vi "函数类型1测试.vi"() -> ()   [LabVIEW 2010]
uses:
  全局量/试验配置信息.vi
  全局量/全局_配置.vi
panel:
  out "D_IN_1":string[][](table) caption="表格"
  in  "加载文件名称":string
  out "配置文件路径":path
  out "配置文件目录":path
  in  "加载配置文件列表":u16(ring)
  in  "同步_1":i32
  in  "数组_反馈值":dbl[][](array[numeric])
  in  "第几个数据":i32
  in  "第几组数据":i32
  out "数组_AD幅值":sgl[](array[numeric])
  out "数组_DSP幅值":sgl[](array[numeric])
  in  "数组_设定值":dbl[][](array[numeric])
  in  "数组_选择":bool[](array[boolean])
  out "light_32":bool
  out "light_31":bool
  out "light_30":bool
  out "light_29":bool
  out "light_28":bool
  out "light_27":bool
  out "light_26":bool
  out "light_25":bool
  out "light_24":bool
  out "light_23":bool
  out "light_22":bool
  out "light_21":bool
  out "light_20":bool
  out "light_19":bool
  out "light_18":bool
  out "light_17":bool
  out "Analog_back":string[][](table) caption="表格"
  in  "A_32":bool
  in  "A_31":bool
  in  "A_30":bool
  in  "A_29":bool
  in  "A_28":bool
  in  "A_27":bool
  in  "A_26":bool
  in  "A_25":bool
  in  "A_24":bool
  in  "A_23":bool
  in  "A_22":bool
  in  "A_21":bool
  in  "A_20":bool
  in  "A_19":bool
  in  "A_18":bool
  in  "A_17":bool
  out "合格？":bool[][](array[boolean])
  out "测试结论":string
  out "light_16":bool
  out "light_15":bool
  out "light_14":bool
  out "light_13":bool
  out "light_12":bool
  out "light_11":bool
  out "light_10":bool
  out "light_9":bool
  out "light_8":bool
  out "light_7":bool
  out "light_6":bool
  out "light_5":bool
  out "light_4":bool
  out "light_3":bool
  out "light_2":bool
  out "light_1":bool
  out "退出？":bool
  in  "btn_反选":bool
  in  "btn_全选":bool
  in  "A_16":bool
  in  "A_15":bool
  in  "A_14":bool
  in  "A_13":bool
  in  "A_12":bool
  in  "A_11":bool
  in  "A_10":bool
  in  "A_9":bool
  in  "A_8":bool
  in  "A_7":bool
  in  "A_6":bool
  in  "A_5":bool
  in  "A_4":bool
  in  "A_3":bool
  in  "A_2":bool
  in  "A_1":bool
  in  "btn_取消":bool
  in  "btn_开始测试":bool
  in  "Analog_IN":string[][](table) caption="表格"
  out "Analog_WC":string[][](table) caption="表格"
  # "模拟量选择及输入值（V）"
  # "模拟量反馈值（V）"
  # "模拟量误差值（%）"
  # "加载配置文件："
  # "测试结论："
  # "从0开始"
  # "从1开始,第0列没有使用"
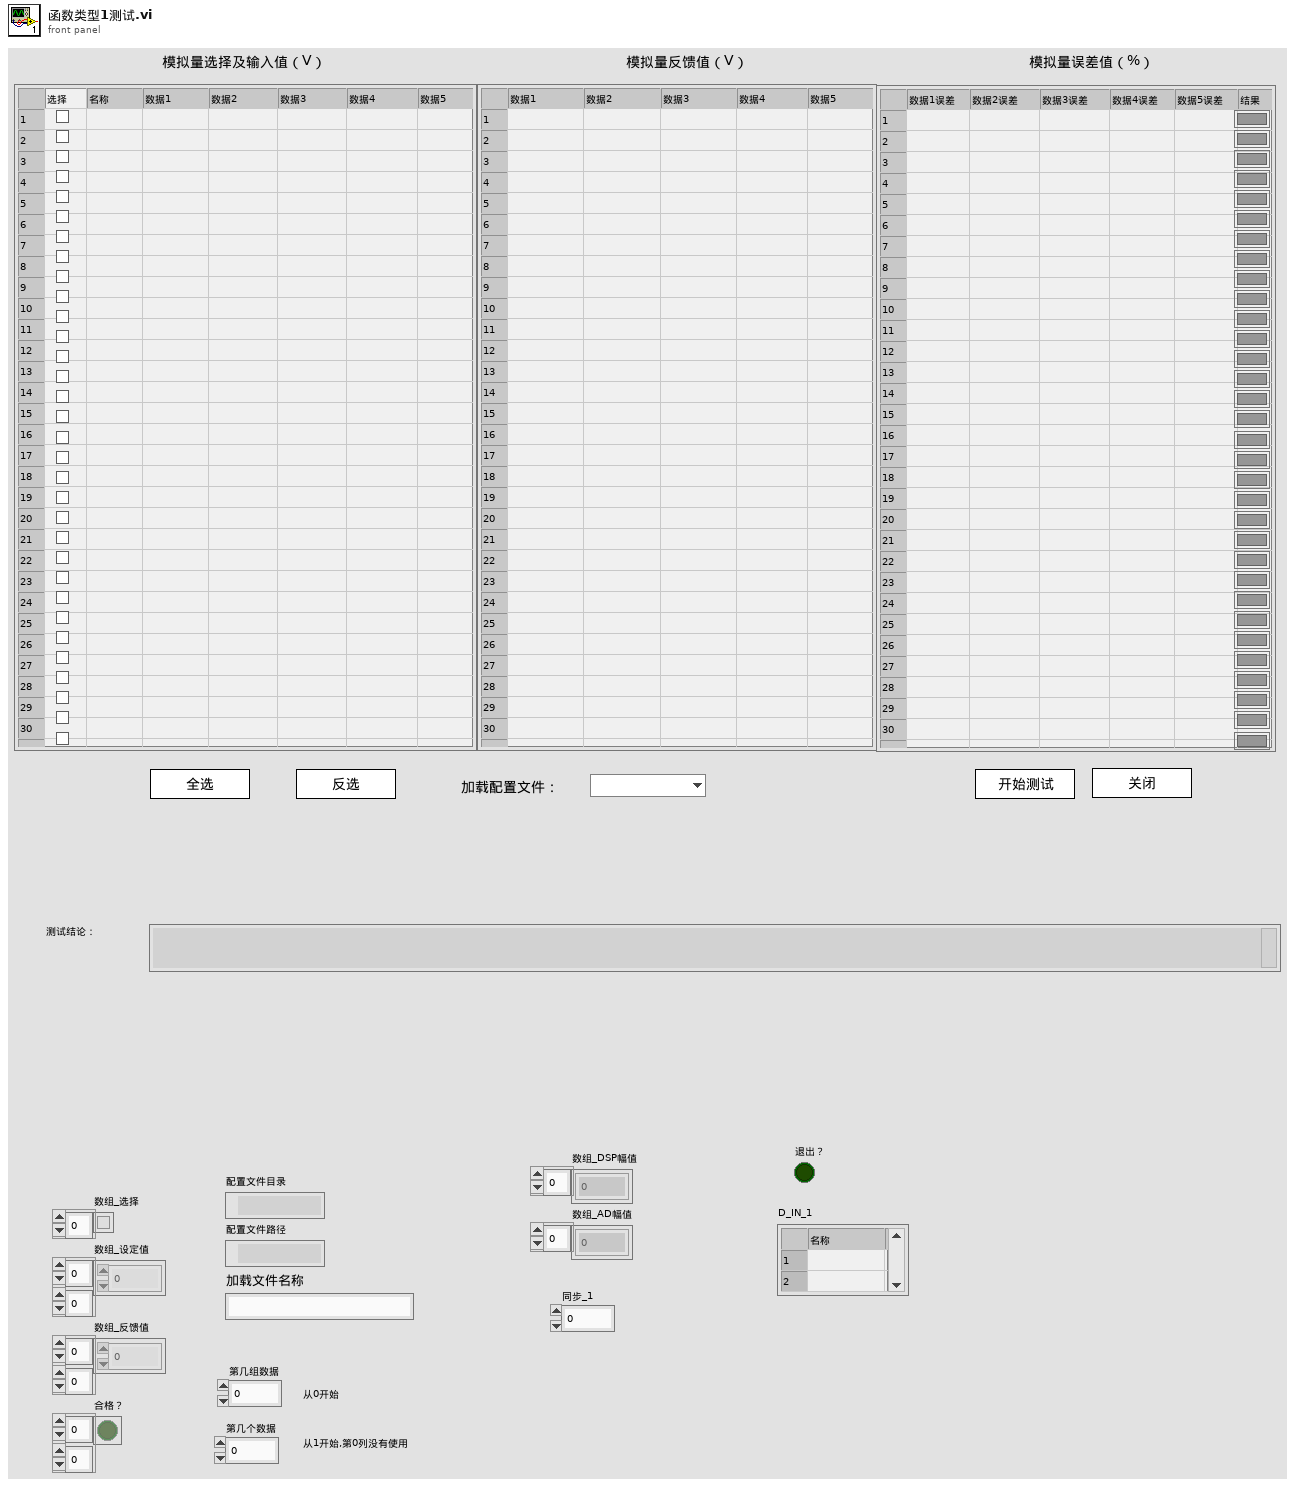
[diagram p1: front panel]
types:
  T1 = enum8{"Enabled", "Disabled", "Disabled and Grayed Out"}
  T2 = cluster{"数字量输入信号路数":u32, "数字量输出信号路数":u32, "DSP模拟量输入信号路数":u32, "DSP模拟量输入信号幅值":u32, "AD模拟量输入信号路数":u32, "AD模拟量输入信号幅值":u32, "RS232端口":u32, "RS232通信路数":u32, "RS232波特率":u32, "RS485端口":u32, "RS485通信路数":u32, "RS485波特率":u32, "CAN通信端口":string, "CAN波特率":u32, "以太网选择?":bool, "控制板IP":string, "以太网端口":u32}
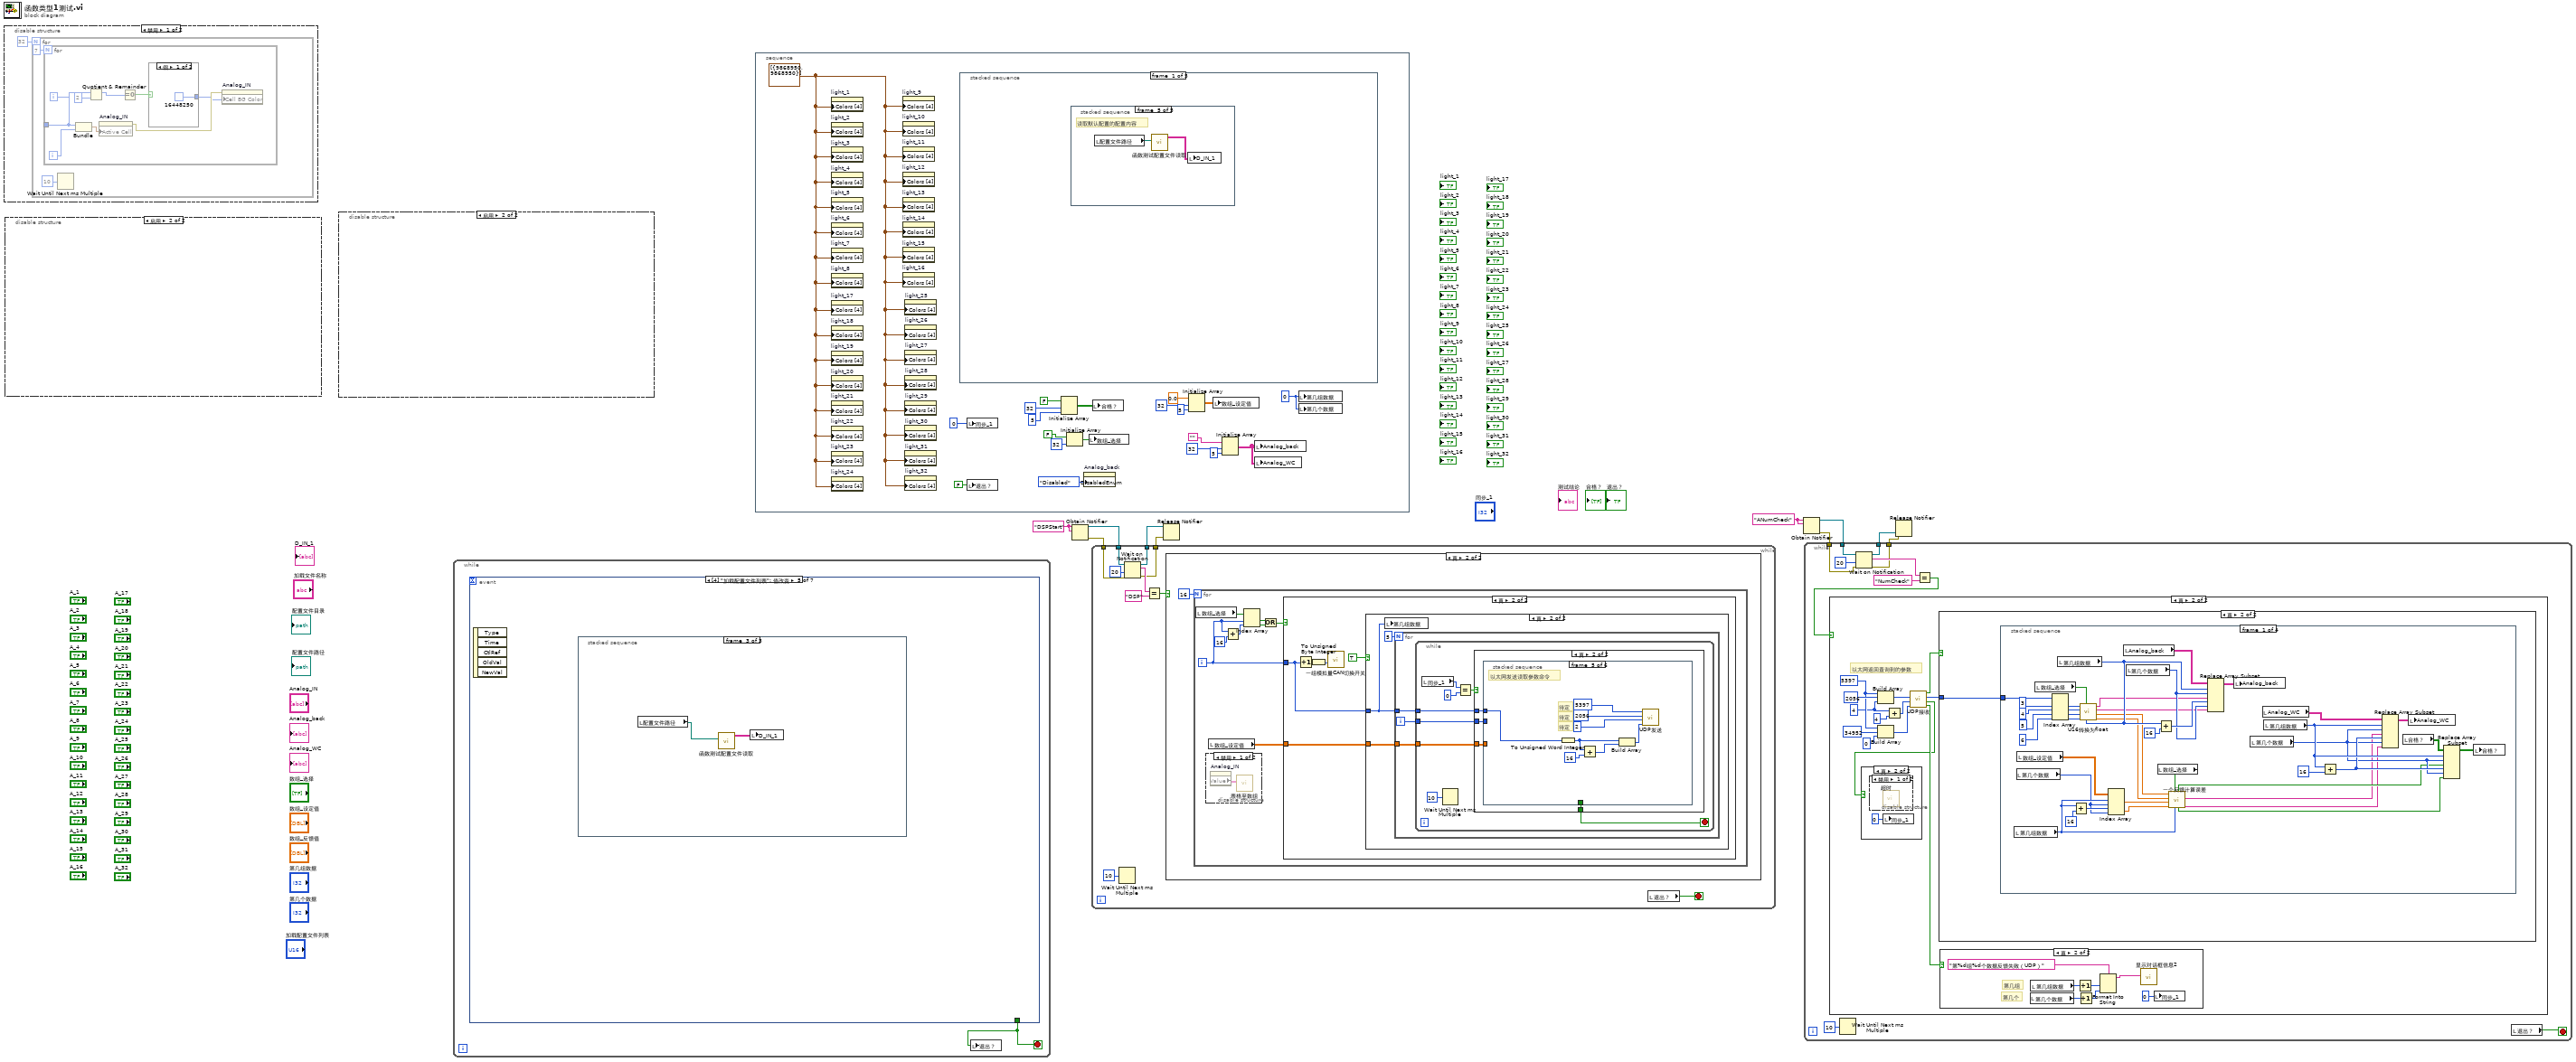
[diagram p0: block diagram]
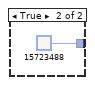
[diagram p2: hidden frame]
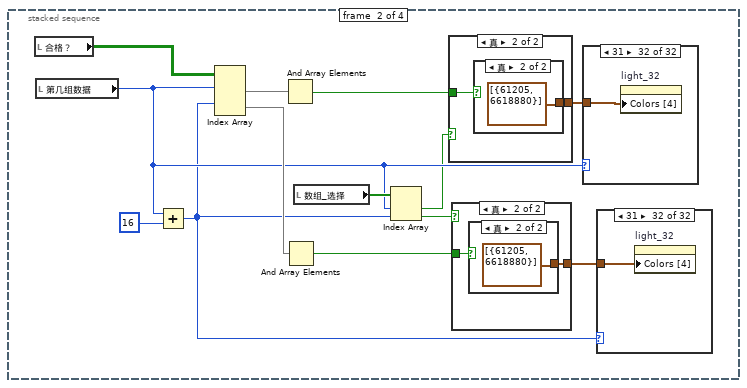
[diagram p9: hidden frame]
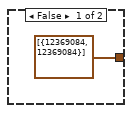
[diagram p10: hidden frame]
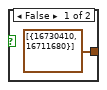
[diagram p11: hidden frame]
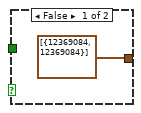
[diagram p12: hidden frame]
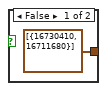
[diagram p13: hidden frame]
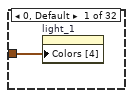
[diagram p14: hidden frame]
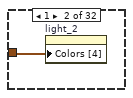
[diagram p15: hidden frame]
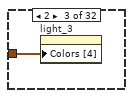
[diagram p16: hidden frame]
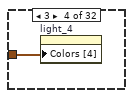
[diagram p17: hidden frame]
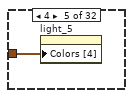
[diagram p18: hidden frame]
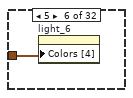
[diagram p19: hidden frame]
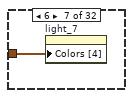
[diagram p20: hidden frame]
diagram:
  w5 = "ANumCheck" ("名称（未命名）")
  w8 = "DSPStart" ("名称（未命名）")
  n1 = disable-structure shown="禁用" {
    frame Disabled {
      n2 = for {
        N: 32 -> [_]
        i -> [w13]
        n3 = for {
          N: 7 -> [_]
          tunnel: w13 -> [w21]
          i -> [w15]
          n4 = Bundle(w21, w15) -> (w18:cluster{i32, i32})  [unwired: 1 in]
          n5 = Quotient & Remainder(x=w21, y=2) -> (x-y*floor(x/y)=w19:i32)  [unwired: 1 out]
          n6 = property on="Analog_IN" class="Tbl (严格)"("Active Cell"=w18) -> (error out=w17:errorcluster)  [unwired: 2 in, 1 out]
          n7 = Equal To 0?(x=w19) -> (x = 0?=w22:bool)
          n8 = case shown="假" w22 {
            tunnel: [u32 16448250 u32 15723488] -> w16
            frame False {
            }
            frame True {
            }
          }
          n9 = property on="Analog_IN" class="Tbl (严格)"(error in=w17, "Cell BG Color"=w16) -> ()  [unwired: 1 in, 2 out]
        }
        n10 = Wait Until Next ms Multiple(millisecond multiple=u32 10 ("毫秒倍数")) -> ()  [unwired: 1 out]
      }
    }
    frame Enabled {
    }
  }
  n11 = disable-structure shown="启用" {
    frame Disabled {
      n12 = for {
        N: 32 -> [_]
        i -> [w26]
        n13 = for {
          N: 7 -> [_]
          tunnel: w26 -> [w29]
          i -> [w30]
          n14 = Bundle(w29, w30) -> (w33:cluster{i32, i32})  [unwired: 1 in]
          n15 = property on="Analog_IN" class="Tbl (严格)"("Active Cell"=w33) -> (error out=w31:errorcluster)  [unwired: 2 in, 1 out]
          n16 = property on="Analog_IN" class="Tbl (严格)"(error in=w31, "Justify"=enum16{"Left", "Center", "Right"}."Left" ("活动单元格:单元格对齐")) -> ()  [unwired: 1 in, 2 out]
        }
        n17 = Wait Until Next ms Multiple(millisecond multiple=u32 10 ("毫秒倍数")) -> ()  [unwired: 1 out]
      }
    }
    frame Enabled {
    }
  }
  n18 = disable-structure shown="启用" {
    frame Disabled {
      n19 = for {
        N: 32 -> [_]
        i -> [w39]
        n20 = Wait Until Next ms Multiple(millisecond multiple=u32 10 ("毫秒倍数")) -> ()  [unwired: 1 out]
        n21 = Bundle(w39, 1) -> (w38:cluster{i32, i32})  [unwired: 1 in]
        n22 = property on="Analog_IN" class="Tbl (严格)"("Active Cell"=w38) -> (error out=w35:errorcluster)  [unwired: 2 in, 1 out]
        n23 = property on="Analog_IN" class="Tbl (严格)"(error in=w35, "DisabledEnum"=T1."Enabled" ("禁用")) -> ()  [unwired: 1 in, 2 out]
      }
    }
    frame Enabled {
    }
  }
  n24 = while {
    stop <- w41 stop-if-true
    n25 = event shown="[4] \"加载配置文件列表\": 值改变" {
      selector: _ -> [_ _ _ _ _ _ _]
      dyn-events: _ -> [_ _ _ _ _ _ _]
      timeout: _ -> [_ _ _ _ _ _ _]
      tunnel: [_ TRUE TRUE _ _ _ _] -> w41
      event Timeout {
        n26 = event-data() -> ()  [unwired: 1 in, 2 out]
      }
      event Panel Close {
        n27 = event-data() -> ()  [unwired: 1 in, 3 out]
      }
      event "btn_取消": Value Change {
        n28 = event-data() -> ()  [unwired: 1 in, 5 out]
      }
      event "btn_开始测试": Value Change {
        n29 = event-data() -> ()  [unwired: 1 in, 5 out]
        n30 = stacked-sequence {
          frame #0 {
            w48 = 0 ("第几组数据")
            n31 = local read "Analog_IN"() -> (w54:string[][])
            n32 = Delete From Array(array=w54, length=1 ("长度"), index (col)=0 ("禁用的索引 (列)")) -> (array with subset deleted=w46:string[][])  [unwired: 1 in, 1 out]
            n33 = Delete From Array(array=w46, length=1 ("长度"), index (col)=0 ("禁用的索引 (列)")) -> (array with subset deleted=w44:string[][])  [unwired: 1 in, 1 out]
            n34 = for {
              N: 32 -> [_]
              tunnel: w44 -> [w57] mode=indexing
              tunnel: [w56] -> w53 mode=indexing
              n35 = for {
                N: 5 -> [_]
                tunnel: w57 -> [w59] mode=indexing
                tunnel: [w58] -> w56 mode=indexing
                n36 = Fract/Exp String To Number(string=w59) -> (number=w58:dbl)  [unwired: 3 in, 1 out]
              }
            }
            n37 = local write "第几组数据"(w48) -> ()
            n38 = local write "第几个数据"(w48) -> ()
            n39 = local write "同步_1"(0 ("同步_2")) -> ()
            n40 = local write "数组_设定值"(w53) -> ()
          }
          frame #1 {
            n41 = local read "Analog_back"() -> (w62:string[][])
            n42 = local read "Analog_WC"() -> (w61:string[][])
            n43 = for {
              tunnel: w61 -> [w98] mode=indexing
              i -> [w97]
              n44 = for {
                tunnel: w98 -> [_] mode=indexing
                tunnel: w97 -> [w102]
                i -> [w101]
                n45 = local read "Analog_WC"() -> (w103:string[][])
                n46 = Replace Array Subset(array=w103, new element="", index (row)=w102, index (col)=w101) -> (w99:string[][])
                n47 = local write "Analog_WC"(w99) -> ()
              }
            }
            n48 = for {
              tunnel: w62 -> [w105] mode=indexing
              i -> [w104]
              n49 = for {
                tunnel: w105 -> [_] mode=indexing
                tunnel: w104 -> [w109]
                i -> [w108]
                n50 = local read "Analog_back"() -> (w110:string[][])
                n51 = Replace Array Subset(array=w110, new element="", index (row)=w109, index (col)=w108) -> (w106:string[][])
                n52 = local write "Analog_back"(w106) -> ()
              }
            }
            n53 = for {
              N: 32 -> [_]
              i -> [w64]
              n54 = case shown="31" w64 {
                tunnel: cluster{u32, u32}[] [{9868950, 9868950}] -> [w65 w66 w67 w68 w69 w70 w71 w72 w73 w74 w75 w76 w77 w78 w79 w80 w81 w82 w83 w84 w85 w86 w87 w88 w89 w90 w91 w92 w93 w94 w95 w96]
                frame 0, Default {
                  n55 = property on="light_1" class="Bool (严格)"("Colors [4]"=w65) -> ()  [unwired: 2 in, 2 out]
                }
                frame 1 {
                  n56 = property on="light_2" class="Bool (严格)"("Colors [4]"=w66) -> ()  [unwired: 2 in, 2 out]
                }
                frame 2 {
                  n57 = property on="light_3" class="Bool (严格)"("Colors [4]"=w67) -> ()  [unwired: 2 in, 2 out]
                }
                frame 3 {
                  n58 = property on="light_4" class="Bool (严格)"("Colors [4]"=w68) -> ()  [unwired: 2 in, 2 out]
                }
                frame 4 {
                  n59 = property on="light_5" class="Bool (严格)"("Colors [4]"=w69) -> ()  [unwired: 2 in, 2 out]
                }
                frame 5 {
                  n60 = property on="light_6" class="Bool (严格)"("Colors [4]"=w70) -> ()  [unwired: 2 in, 2 out]
                }
                frame 6 {
                  n61 = property on="light_7" class="Bool (严格)"("Colors [4]"=w71) -> ()  [unwired: 2 in, 2 out]
                }
                frame 7 {
                  n62 = property on="light_8" class="Bool (严格)"("Colors [4]"=w72) -> ()  [unwired: 2 in, 2 out]
                }
                frame 8 {
                  n63 = property on="light_9" class="Bool (严格)"("Colors [4]"=w73) -> ()  [unwired: 2 in, 2 out]
                }
                frame 9 {
                  n64 = property on="light_10" class="Bool (严格)"("Colors [4]"=w74) -> ()  [unwired: 2 in, 2 out]
                }
                frame 10 {
                  n65 = property on="light_11" class="Bool (严格)"("Colors [4]"=w75) -> ()  [unwired: 2 in, 2 out]
                }
                frame 11 {
                  n66 = property on="light_12" class="Bool (严格)"("Colors [4]"=w76) -> ()  [unwired: 2 in, 2 out]
                }
                frame 12 {
                  n67 = property on="light_13" class="Bool (严格)"("Colors [4]"=w77) -> ()  [unwired: 2 in, 2 out]
                }
                frame 13 {
                  n68 = property on="light_14" class="Bool (严格)"("Colors [4]"=w78) -> ()  [unwired: 2 in, 2 out]
                }
                frame 14 {
                  n69 = property on="light_15" class="Bool (严格)"("Colors [4]"=w79) -> ()  [unwired: 2 in, 2 out]
                }
                frame 15 {
                  n70 = property on="light_16" class="Bool (严格)"("Colors [4]"=w80) -> ()  [unwired: 2 in, 2 out]
                }
                frame 16 {
                  n71 = property on="light_17" class="Bool (严格)"("Colors [4]"=w81) -> ()  [unwired: 2 in, 2 out]
                }
                frame 17 {
                  n72 = property on="light_18" class="Bool (严格)"("Colors [4]"=w82) -> ()  [unwired: 2 in, 2 out]
                }
                frame 18 {
                  n73 = property on="light_19" class="Bool (严格)"("Colors [4]"=w83) -> ()  [unwired: 2 in, 2 out]
                }
                frame 19 {
                  n74 = property on="light_20" class="Bool (严格)"("Colors [4]"=w84) -> ()  [unwired: 2 in, 2 out]
                }
                frame 20 {
                  n75 = property on="light_21" class="Bool (严格)"("Colors [4]"=w85) -> ()  [unwired: 2 in, 2 out]
                }
                frame 21 {
                  n76 = property on="light_22" class="Bool (严格)"("Colors [4]"=w86) -> ()  [unwired: 2 in, 2 out]
                }
                frame 22 {
                  n77 = property on="light_23" class="Bool (严格)"("Colors [4]"=w87) -> ()  [unwired: 2 in, 2 out]
                }
                frame 23 {
                  n78 = property on="light_24" class="Bool (严格)"("Colors [4]"=w88) -> ()  [unwired: 2 in, 2 out]
                }
                frame 24 {
                  n79 = property on="light_25" class="Bool (严格)"("Colors [4]"=w89) -> ()  [unwired: 2 in, 2 out]
                }
                frame 25 {
                  n80 = property on="light_26" class="Bool (严格)"("Colors [4]"=w90) -> ()  [unwired: 2 in, 2 out]
                }
                frame 26 {
                  n81 = property on="light_27" class="Bool (严格)"("Colors [4]"=w91) -> ()  [unwired: 2 in, 2 out]
                }
                frame 27 {
                  n82 = property on="light_28" class="Bool (严格)"("Colors [4]"=w92) -> ()  [unwired: 2 in, 2 out]
                }
                frame 28 {
                  n83 = property on="light_29" class="Bool (严格)"("Colors [4]"=w93) -> ()  [unwired: 2 in, 2 out]
                }
                frame 29 {
                  n84 = property on="light_30" class="Bool (严格)"("Colors [4]"=w94) -> ()  [unwired: 2 in, 2 out]
                }
                frame 30 {
                  n85 = property on="light_31" class="Bool (严格)"("Colors [4]"=w95) -> ()  [unwired: 2 in, 2 out]
                }
                frame 31 {
                  n86 = property on="light_32" class="Bool (严格)"("Colors [4]"=w96) -> ()  [unwired: 2 in, 2 out]
                }
              }
            }
          }
          frame #2 {
            n87 = for {
              N: 32 -> [_]
              i -> [w113]
              n88 = disable-structure shown="禁用" {
                frame Disabled {
                  n89 = Wait Until Next ms Multiple(millisecond multiple=u32 10 ("毫秒倍数")) -> ()  [unwired: 1 out]
                }
                frame Enabled {
                }
              }
              n90 = for {
                N: 6 -> [_]
                tunnel: w113 -> [w121]
                i -> [w118]
                n91 = Bundle(w121, w118) -> (w117:cluster{i32, i32})  [unwired: 1 in]
                n92 = Quotient & Remainder(x=w121, y=2) -> (x-y*floor(x/y)=w119:i32)  [unwired: 1 out]
                n93 = property on="Analog_WC" class="Tbl (严格)"("Active Cell"=w117) -> (error out=w116:errorcluster)  [unwired: 2 in, 1 out]
                n94 = Equal To 0?(x=w119) -> (x = 0?=w122:bool)
                n95 = case shown="假" w122 {
                  tunnel: [u32 16448250 u32 15723488] -> w115
                  frame False {
                  }
                  frame True {
                  }
                }
                n96 = property on="Analog_WC" class="Tbl (严格)"(error in=w116, "Cell BG Color"=w115) -> ()  [unwired: 1 in, 2 out]
              }
            }
          }
          frame #3 {
            n97 = local read "A_10"() -> (w153:bool)
            n98 = local read "A_11"() -> (w152:bool)
            n99 = local read "A_12"() -> (w151:bool)
            n100 = local read "A_13"() -> (w150:bool)
            n101 = local read "A_14"() -> (w149:bool)
            n102 = local read "A_15"() -> (w148:bool)
            n103 = local read "A_16"() -> (w147:bool)
            n104 = local read "A_17"() -> (w146:bool)
            n105 = local read "A_18"() -> (w145:bool)
            n106 = local read "A_19"() -> (w144:bool)
            n107 = local read "A_20"() -> (w143:bool)
            n108 = local read "A_21"() -> (w142:bool)
            n109 = local read "A_22"() -> (w141:bool)
            n110 = local read "A_23"() -> (w140:bool)
            n111 = local read "A_24"() -> (w139:bool)
            n112 = local read "A_25"() -> (w138:bool)
            n113 = local read "A_26"() -> (w137:bool)
            n114 = local read "A_27"() -> (w136:bool)
            n115 = local read "A_28"() -> (w135:bool)
            n116 = local read "A_29"() -> (w134:bool)
            n117 = local read "A_30"() -> (w133:bool)
            n118 = local read "A_31"() -> (w132:bool)
            n119 = local read "A_32"() -> (w131:bool)
            n120 = local read "A_1"() -> (w162:bool)
            n121 = local read "A_2"() -> (w161:bool)
            n122 = local read "A_3"() -> (w160:bool)
            n123 = local read "A_4"() -> (w159:bool)
            n124 = local read "A_5"() -> (w158:bool)
            n125 = local read "A_6"() -> (w157:bool)
            n126 = local read "A_7"() -> (w156:bool)
            n127 = local read "A_8"() -> (w155:bool)
            n128 = local read "A_9"() -> (w154:bool)
            n129 = Build Array(w162, w161, w160, w159, w158, w157, w156, w155, w154, w153, w152, w151, w150, w149, w148, w147, w146, w145, w144, w143, w142, w141, w140, w139, w138, w137, w136, w135, w134, w133, w132, w131) -> (w125:bool[])
            n130 = Or Array Elements(Boolean array=w125) -> (logical OR=w130:bool)
            n131 = case shown="真" w130 {
              frame False {
                n132 = call "显示对话框信息"() -> ()  [unwired: 10 in, 2 out]
              }
              frame True {
                w164 = "DSPStart" ("名称（未命名）")
                n133 = Obtain Notifier(name (unnamed)=w164, notification data type=w164) -> (notifier out=w163:refnum<notifier>)  [unwired: 2 in, 2 out]
                n134 = Send Notification(notification="DSP" ("通知"), notifier=w163) -> ()  [unwired: 1 in, 2 out]
              }
            }
            n135 = local write "数组_选择"(w125) -> ()
            n136 = Initialize Array(FALSE, 32 ("维数大小"), 5 ("维数大小")) -> (w126:bool[][])
            n137 = local write "合格？"(w126) -> ()
          }
        }
      }
      event "加载配置文件列表": Value Change {
        n138 = event-data() -> ()  [unwired: 1 in, 5 out]
        n139 = stacked-sequence {
          frame #0 {
            n140 = property on="加载配置文件列表" class="Ring (严格)"() -> ("RingText.Text"=w166:string)  [unwired: 2 in, 2 out]
            n141 = local write "加载文件名称"(w166) -> ()
          }
          frame #1 {
            n142 = local read "配置文件目录"() -> (w169:path)
            n143 = property on="加载文件名称" class="Str"() -> ("Text.Text"=w167:string)  [unwired: 2 in, 2 out]
            n144 = Build Path(base path=w169, name or relative path=w167) -> (appended path=w168:path)
            n145 = local write "配置文件路径"(w168) -> ()
          }
          frame #2 {
            n146 = local read "配置文件路径"() -> (w171:path)
            n147 = call "函数测试配置文件读取.vi"("配置文件路径"=w171) -> ("D_IN_1"=w170:string[][])  [unwired: 6 in, 3 out]
            n148 = local write "D_IN_1"(w170) -> ()
          }
        }
      }
      event "btn_全选": Value Change {
        w172 = TRUE ("单选_AD_1")
        n149 = event-data() -> ()  [unwired: 1 in, 5 out]
        n150 = local write "A_1"(w172) -> ()
        n151 = local write "A_2"(w172) -> ()
        n152 = local write "A_3"(w172) -> ()
        n153 = local write "A_4"(w172) -> ()
        n154 = local write "A_5"(w172) -> ()
        n155 = local write "A_6"(w172) -> ()
        n156 = local write "A_7"(w172) -> ()
        n157 = local write "A_8"(w172) -> ()
        n158 = local write "A_9"(w172) -> ()
        n159 = local write "A_10"(w172) -> ()
        n160 = local write "A_11"(w172) -> ()
        n161 = local write "A_12"(w172) -> ()
        n162 = local write "A_13"(w172) -> ()
        n163 = local write "A_14"(w172) -> ()
        n164 = local write "A_15"(w172) -> ()
        n165 = local write "A_16"(w172) -> ()
        n166 = local write "A_17"(w172) -> ()
        n167 = local write "A_18"(w172) -> ()
        n168 = local write "A_19"(w172) -> ()
        n169 = local write "A_20"(w172) -> ()
        n170 = local write "A_21"(w172) -> ()
        n171 = local write "A_22"(w172) -> ()
        n172 = local write "A_23"(w172) -> ()
        n173 = local write "A_24"(w172) -> ()
        n174 = local write "A_25"(w172) -> ()
        n175 = local write "A_26"(w172) -> ()
        n176 = local write "A_27"(w172) -> ()
        n177 = local write "A_28"(w172) -> ()
        n178 = local write "A_29"(w172) -> ()
        n179 = local write "A_30"(w172) -> ()
        n180 = local write "A_31"(w172) -> ()
        n181 = local write "A_32"(w172) -> ()
      }
      event "btn_反选": Value Change {
        n182 = event-data() -> ()  [unwired: 1 in, 5 out]
        n183 = local read "A_17"() -> (w204:bool)
        n184 = local read "A_18"() -> (w202:bool)
        n185 = local read "A_19"() -> (w200:bool)
        n186 = local read "A_20"() -> (w198:bool)
        n187 = local read "A_21"() -> (w196:bool)
        n188 = local read "A_22"() -> (w194:bool)
        n189 = local read "A_23"() -> (w192:bool)
        n190 = local read "A_24"() -> (w190:bool)
        n191 = local read "A_25"() -> (w188:bool)
        n192 = local read "A_26"() -> (w186:bool)
        n193 = local read "A_27"() -> (w184:bool)
        n194 = local read "A_28"() -> (w182:bool)
        n195 = local read "A_29"() -> (w180:bool)
        n196 = local read "A_30"() -> (w178:bool)
        n197 = local read "A_31"() -> (w176:bool)
        n198 = local read "A_32"() -> (w174:bool)
        n199 = local read "A_1"() -> (w236:bool)
        n200 = local read "A_2"() -> (w234:bool)
        n201 = local read "A_3"() -> (w233:bool)
        n202 = local read "A_4"() -> (w232:bool)
        n203 = local read "A_5"() -> (w231:bool)
        n204 = local read "A_6"() -> (w230:bool)
        n205 = local read "A_7"() -> (w229:bool)
        n206 = local read "A_8"() -> (w228:bool)
        n207 = local read "A_9"() -> (w227:bool)
        n208 = local read "A_10"() -> (w226:bool)
        n209 = local read "A_11"() -> (w225:bool)
        n210 = local read "A_12"() -> (w224:bool)
        n211 = local read "A_13"() -> (w223:bool)
        n212 = local read "A_14"() -> (w222:bool)
        n213 = local read "A_15"() -> (w221:bool)
        n214 = local read "A_16"() -> (w220:bool)
        n215 = Not(x=w236) -> (.not. x?=w235:bool)
        n216 = Not(x=w234) -> (.not. x?=w205:bool)
        n217 = Not(x=w233) -> (.not. x?=w206:bool)
        n218 = Not(x=w232) -> (.not. x?=w207:bool)
        n219 = Not(x=w231) -> (.not. x?=w208:bool)
        n220 = Not(x=w230) -> (.not. x?=w209:bool)
        n221 = Not(x=w229) -> (.not. x?=w210:bool)
        n222 = Not(x=w228) -> (.not. x?=w211:bool)
        n223 = Not(x=w227) -> (.not. x?=w212:bool)
        n224 = Not(x=w226) -> (.not. x?=w213:bool)
        n225 = Not(x=w225) -> (.not. x?=w214:bool)
        n226 = Not(x=w224) -> (.not. x?=w215:bool)
        n227 = Not(x=w223) -> (.not. x?=w216:bool)
        n228 = Not(x=w222) -> (.not. x?=w217:bool)
        n229 = Not(x=w221) -> (.not. x?=w218:bool)
        n230 = Not(x=w220) -> (.not. x?=w219:bool)
        n231 = Not(x=w204) -> (.not. x?=w203:bool)
        n232 = Not(x=w202) -> (.not. x?=w201:bool)
        n233 = Not(x=w200) -> (.not. x?=w199:bool)
        n234 = Not(x=w198) -> (.not. x?=w197:bool)
        n235 = Not(x=w196) -> (.not. x?=w195:bool)
        n236 = Not(x=w194) -> (.not. x?=w193:bool)
        n237 = Not(x=w192) -> (.not. x?=w191:bool)
        n238 = Not(x=w190) -> (.not. x?=w189:bool)
        n239 = Not(x=w188) -> (.not. x?=w187:bool)
        n240 = Not(x=w186) -> (.not. x?=w185:bool)
        n241 = Not(x=w184) -> (.not. x?=w183:bool)
        n242 = Not(x=w182) -> (.not. x?=w181:bool)
        n243 = Not(x=w180) -> (.not. x?=w179:bool)
        n244 = Not(x=w178) -> (.not. x?=w177:bool)
        n245 = Not(x=w176) -> (.not. x?=w175:bool)
        n246 = Not(x=w174) -> (.not. x?=w173:bool)
        n247 = local write "A_1"(w235) -> ()
        n248 = local write "A_2"(w205) -> ()
        n249 = local write "A_3"(w206) -> ()
        n250 = local write "A_4"(w207) -> ()
        n251 = local write "A_5"(w208) -> ()
        n252 = local write "A_6"(w209) -> ()
        n253 = local write "A_7"(w210) -> ()
        n254 = local write "A_8"(w211) -> ()
        n255 = local write "A_9"(w212) -> ()
        n256 = local write "A_10"(w213) -> ()
        n257 = local write "A_11"(w214) -> ()
        n258 = local write "A_12"(w215) -> ()
        n259 = local write "A_13"(w216) -> ()
        n260 = local write "A_14"(w217) -> ()
        n261 = local write "A_15"(w218) -> ()
        n262 = local write "A_16"(w219) -> ()
        n263 = local write "A_17"(w203) -> ()
        n264 = local write "A_18"(w201) -> ()
        n265 = local write "A_19"(w199) -> ()
        n266 = local write "A_20"(w197) -> ()
        n267 = local write "A_21"(w195) -> ()
        n268 = local write "A_22"(w193) -> ()
        n269 = local write "A_23"(w191) -> ()
        n270 = local write "A_24"(w189) -> ()
        n271 = local write "A_25"(w187) -> ()
        n272 = local write "A_26"(w185) -> ()
        n273 = local write "A_27"(w183) -> ()
        n274 = local write "A_28"(w181) -> ()
        n275 = local write "A_29"(w179) -> ()
        n276 = local write "A_30"(w177) -> ()
        n277 = local write "A_31"(w175) -> ()
        n278 = local write "A_32"(w173) -> ()
      }
    }
    n279 = local write "退出？"(w41) -> ()
  }
  n280 = stacked-sequence {
    frame #0 {
      w237 = 0 ("第几组数据")
      w252 = cluster{u32, u32}[] [{9868950, 9868950}]
      n281 = property on="light_1" class="Bool (严格)"("Colors [4]"=w252) -> ()  [unwired: 2 in, 2 out]
      n282 = property on="light_2" class="Bool (严格)"("Colors [4]"=w252) -> ()  [unwired: 2 in, 2 out]
      n283 = property on="light_3" class="Bool (严格)"("Colors [4]"=w252) -> ()  [unwired: 2 in, 2 out]
      n284 = property on="light_4" class="Bool (严格)"("Colors [4]"=w252) -> ()  [unwired: 2 in, 2 out]
      n285 = property on="light_5" class="Bool (严格)"("Colors [4]"=w252) -> ()  [unwired: 2 in, 2 out]
      n286 = property on="light_6" class="Bool (严格)"("Colors [4]"=w252) -> ()  [unwired: 2 in, 2 out]
      n287 = property on="light_7" class="Bool (严格)"("Colors [4]"=w252) -> ()  [unwired: 2 in, 2 out]
      n288 = property on="light_8" class="Bool (严格)"("Colors [4]"=w252) -> ()  [unwired: 2 in, 2 out]
      n289 = property on="light_17" class="Bool (严格)"("Colors [4]"=w252) -> ()  [unwired: 2 in, 2 out]
      n290 = property on="light_18" class="Bool (严格)"("Colors [4]"=w252) -> ()  [unwired: 2 in, 2 out]
      n291 = property on="light_19" class="Bool (严格)"("Colors [4]"=w252) -> ()  [unwired: 2 in, 2 out]
      n292 = property on="light_20" class="Bool (严格)"("Colors [4]"=w252) -> ()  [unwired: 2 in, 2 out]
      n293 = property on="light_21" class="Bool (严格)"("Colors [4]"=w252) -> ()  [unwired: 2 in, 2 out]
      n294 = property on="light_22" class="Bool (严格)"("Colors [4]"=w252) -> ()  [unwired: 2 in, 2 out]
      n295 = property on="light_23" class="Bool (严格)"("Colors [4]"=w252) -> ()  [unwired: 2 in, 2 out]
      n296 = property on="light_24" class="Bool (严格)"("Colors [4]"=w252) -> ()  [unwired: 2 in, 2 out]
      n297 = property on="light_9" class="Bool (严格)"("Colors [4]"=w252) -> ()  [unwired: 2 in, 2 out]
      n298 = property on="light_10" class="Bool (严格)"("Colors [4]"=w252) -> ()  [unwired: 2 in, 2 out]
      n299 = property on="light_11" class="Bool (严格)"("Colors [4]"=w252) -> ()  [unwired: 2 in, 2 out]
      n300 = property on="light_12" class="Bool (严格)"("Colors [4]"=w252) -> ()  [unwired: 2 in, 2 out]
      n301 = property on="light_13" class="Bool (严格)"("Colors [4]"=w252) -> ()  [unwired: 2 in, 2 out]
      n302 = property on="light_14" class="Bool (严格)"("Colors [4]"=w252) -> ()  [unwired: 2 in, 2 out]
      n303 = property on="light_15" class="Bool (严格)"("Colors [4]"=w252) -> ()  [unwired: 2 in, 2 out]
      n304 = property on="light_16" class="Bool (严格)"("Colors [4]"=w252) -> ()  [unwired: 2 in, 2 out]
      n305 = property on="light_25" class="Bool (严格)"("Colors [4]"=w252) -> ()  [unwired: 2 in, 2 out]
      n306 = property on="light_26" class="Bool (严格)"("Colors [4]"=w252) -> ()  [unwired: 2 in, 2 out]
      n307 = property on="light_27" class="Bool (严格)"("Colors [4]"=w252) -> ()  [unwired: 2 in, 2 out]
      n308 = property on="light_28" class="Bool (严格)"("Colors [4]"=w252) -> ()  [unwired: 2 in, 2 out]
      n309 = property on="light_29" class="Bool (严格)"("Colors [4]"=w252) -> ()  [unwired: 2 in, 2 out]
      n310 = property on="light_30" class="Bool (严格)"("Colors [4]"=w252) -> ()  [unwired: 2 in, 2 out]
      n311 = property on="light_31" class="Bool (严格)"("Colors [4]"=w252) -> ()  [unwired: 2 in, 2 out]
      n312 = property on="light_32" class="Bool (严格)"("Colors [4]"=w252) -> ()  [unwired: 2 in, 2 out]
      n313 = stacked-sequence {
        frame #0 {
          n314 = stacked-sequence {
            frame #0 {
              # "初始化配置文件路径"
              n315 = VI Library "VI库"() -> (path=w262:path)
              n316 = Strip Path(path=w262) -> (stripped path=w261:path)  [unwired: 1 out]
              n317 = Build Path(base path=w261, name or relative path="config" ("名称或相对路径")) -> (appended path=w259:path)
              n318 = Build Path(base path=w259, name or relative path="函数测试配置文件" ("名称或相对路径")) -> (appended path=w257:path)
              n319 = local write "配置文件目录"(w257) -> ()
            }
            frame #1 {
              # "遍历配置文件目录"
              n320 = local read "配置文件目录"() -> (w263:path)
              n321 = call "罗列目录配置文件.vi"("路径"=w263) -> ("数组"=w264:string[])  [unwired: 10 in]
              n322 = property on="加载配置文件列表" class="Ring (严格)"("Strings []"=w264) -> ()  [unwired: 2 in, 2 out]
            }
            frame #2 {
              n323 = property on="加载配置文件列表" class="Ring (严格)"() -> ("RingText.Text"=w265:string)  [unwired: 2 in, 2 out]
              n324 = local write "加载文件名称"(w265) -> ()
            }
            frame #3 {
              # "待读取配置文件路径"
              n325 = local read "配置文件目录"() -> (w267:path)
              n326 = property on="加载文件名称" class="Str"() -> ("Text.Text"=w266:string)  [unwired: 2 in, 2 out]
              n327 = Build Path(base path=w267, name or relative path=w266) -> (appended path=w268:path)
              n328 = local write "配置文件路径"(w268) -> ()
            }
            frame #4 {
              # "读取默认配置的配置内容"
              n329 = local read "配置文件路径"() -> (w270:path)
              n330 = call "函数测试配置文件读取.vi"("配置文件路径"=w270) -> ("D_IN_1"=w269:string[][])  [unwired: 6 in, 3 out]
              n331 = local write "D_IN_1"(w269) -> ()
            }
          }
        }
        frame #1 {
          n332 = Initialize Array("", 32 ("维数大小"), 7 ("维数大小")) -> (w280:string[][])
          n333 = Initialize Array(-15.0 ("元素"), 32 ("维数大小")) -> (w274:dbl[])
          n334 = Initialize Array(15.0 ("元素"), 32 ("维数大小")) -> (w279:dbl[])
          n335 = Initialize Array("测试", 32 ("维数大小")) -> (w272:string[])
          n336 = local write "Analog_IN"(w280) -> ()
          n337 = global write "试验配置信息.vi" "min"(w274) -> ()
          n338 = global write "试验配置信息.vi" "Max"(w279) -> ()
          n339 = global write "试验配置信息.vi" "名称"(w272) -> ()
        }
        frame #2 {
          n340 = disable-structure shown="启用" {
            frame Disabled {
              n341 = global read "全局_配置.vi" "BoardConfig"() -> (w288:T2)
              n342 = Unbundle By Name(w288) -> ("DSP模拟量输入信号幅值"=w287:u32, "AD模拟量输入信号幅值"=w286:u32)
              n343 = case shown="1" w286 {
                tunnel: [sgl 3.0 sgl 5.0 sgl 12.0] -> w284
                frame 0, Default {
                }
                frame 1 {
                }
                frame 2 {
                }
              }
              n344 = case shown="2" w287 {
                tunnel: [sgl 3.0 sgl 5.0 sgl 12.0] -> w285
                frame 0, Default {
                }
                frame 1 {
                }
                frame 2 {
                }
              }
              n345 = for {
                N: 5 -> [_]
                tunnel: w285 -> [w310]
                tunnel: w284 -> [w301]
                tunnel: [w299] -> w290 mode=indexing
                tunnel: [w298] -> w289 mode=indexing
                i -> [w313]
                n346 = Multiply(x=sgl 2.0, y=w310) -> (x*y=w308:sgl)
                n347 = Multiply(x=sgl 2.0, y=w301) -> (x*y=w305:sgl)
                n348 = case shown="4" w313 {
                  tunnel: [sgl 0.05 sgl 0.5 sgl 0.75 sgl 0.95 sgl 0.25] -> w300
                  frame 0, Default {
                  }
                  frame 2 {
                  }
                  frame 3 {
                  }
                  frame 4 {
                  }
                  frame 1 {
                  }
                }
                n349 = Multiply(x=w310, y=sgl -1.0) -> (x*y=w311:sgl)
                n350 = Multiply(x=w301, y=sgl -1.0) -> (x*y=w303:sgl)
                n351 = Multiply(x=w300, y=w308) -> (x*y=w307:sgl)
                n352 = Multiply(x=w300, y=w305) -> (x*y=w306:sgl)
                n353 = Add(x=w307, y=w311) -> (x+y=w299:sgl)
                n354 = Add(x=w306, y=w303) -> (x+y=w298:sgl)
              }
              "数组_DSP幅值" <- w290
              "数组_AD幅值" <- w289
            }
            frame Enabled {
              n355 = Initialize Array(sgl 2.0, 5 ("维数大小")) -> (w321:sgl[])
              n356 = local write "数组_DSP幅值"(w321) -> ()
              n357 = local write "数组_AD幅值"(w321) -> ()
            }
          }
        }
        frame #3 {
          n358 = disable-structure shown="禁用" {
            frame Disabled {
              n359 = stacked-sequence {
                frame #0 {
                  n360 = for {
                    N: 16 -> [_]
                    i -> [w323]
                    n361 = local read "数组_DSP幅值"() -> (w324:sgl[])
                    n362 = for {
                      N: 5 -> [_]
                      tunnel: w324 -> [w332] mode=indexing
                      tunnel: w323 -> [w331]
                      i -> [w328]
                      w326 = i16 2 ("精度(6)")
                      n363 = local read "Analog_IN"() -> (w334:string[][])
                      n364 = Number To Fractional String(number=w332, precision (6)=w326) -> (F-format string=w330:string)  [unwired: 2 in]
                      n365 = Add(x=w328, y=w326) -> (x+y=w327:i32)
                      n366 = Replace Array Subset(array=w334, new element=w330, index (row)=w331, index (col)=w327) -> (w333:string[][])
                      n367 = local write "Analog_IN"(w333) -> ()
                      n368 = Wait Until Next ms Multiple(millisecond multiple=u32 2 ("毫秒倍数")) -> ()  [unwired: 1 out]
                    }
                  }
                }
                frame #1 {
                  n369 = for {
                    N: 16 -> [_]
                    i -> [w337]
                    n370 = local read "数组_AD幅值"() -> (w336:sgl[])
                    n371 = for {
                      N: 5 -> [_]
                      tunnel: w336 -> [w347] mode=indexing
                      tunnel: w337 -> [w344]
                      i -> [w341]
                      w340 = i16 2 ("精度(6)")
                      n372 = Add(x=w344, y=16) -> (x+y=w342:i32)
                      n373 = local read "Analog_IN"() -> (w349:string[][])
                      n374 = Add(x=w341, y=w340) -> (x+y=w339:i32)
                      n375 = Number To Fractional String(number=w347, precision (6)=w340) -> (F-format string=w346:string)  [unwired: 2 in]
                      n376 = Replace Array Subset(array=w349, new element=w346, index (row)=w342, index (col)=w339) -> (w348:string[][])
                      n377 = local write "Analog_IN"(w348) -> ()
                      n378 = Wait Until Next ms Multiple(millisecond multiple=u32 2 ("毫秒倍数")) -> ()  [unwired: 1 out]
                    }
                  }
                }
              }
            }
            frame Enabled {
            }
          }
        }
        frame #4 {
          n379 = for {
            N: 32 -> [_]
            i -> [w353]
            w357 = 5 ("num")
            n380 = global read "试验配置信息.vi" "名称"() -> (w356:string[])
            n381 = global read "试验配置信息.vi" "Max"() -> (w360:dbl[])
            n382 = global read "试验配置信息.vi" "min"() -> (w361:dbl[])
            n383 = Index Array(array=w361, index=w353) -> (element=w359:dbl)
            n384 = Index Array(array=w360, index=w353) -> (element=w358:dbl)
            n385 = for {
              N: w357 -> [_]
              tunnel: w353 -> [w371]
              tunnel: w359 -> [w368]
              tunnel: w358 -> [w367]
              tunnel: w357 -> [w366]
              i -> [w362]
              n386 = call "等分取数据.vi"("Max"=w367, "MIN"=w368, "num"=w366) -> ("数据点"=w365:dbl[])  [unwired: 5 in]
              n387 = Add(x=2, y=w362) -> (x+y=w369:i32)
              n388 = local read "Analog_IN"() -> (w373:string[][])
              n389 = Index Array(array=w365, index=w362) -> (element=w364:dbl)
              n390 = Number To Decimal String(number=w364) -> (decimal integer string=w363:string)  [unwired: 1 in]
              n391 = Replace Array Subset(array=w373, new element=w363, index (row)=w371, index (col)=w369) -> (w372:string[][])
              n392 = local write "Analog_IN"(w372) -> ()
            }
            n393 = Index Array(array=w356, index=w353) -> (element=w351:string)
            n394 = local read "Analog_IN"() -> (w354:string[][])
            n395 = Replace Array Subset(array=w354, new element=w351, index (row)=w353, index (col)=1) -> (w355:string[][])
            n396 = local write "Analog_IN"(w355) -> ()
          }
        }
      }
      n397 = local write "同步_1"(0 ("同步_2")) -> ()
      n398 = local write "退出？"(FALSE ("退出？")) -> ()
      n399 = Initialize Array(FALSE, 32 ("维数大小"), 5 ("维数大小")) -> (w253:bool[][])
      n400 = Initialize Array(FALSE, 32 ("维数大小")) -> (w241:bool[])
      n401 = property on="Analog_back" class="Tbl (严格)"("DisabledEnum"=T1."Disabled" ("禁用")) -> ()  [unwired: 2 in, 2 out]
      n402 = local write "数组_选择"(w241) -> ()
      n403 = local write "合格？"(w253) -> ()
      n404 = Initialize Array(0.0, 32 ("维数大小"), 5 ("维数大小")) -> (w244:dbl[][])
      n405 = local write "数组_设定值"(w244) -> ()
      n406 = Initialize Array("", 32 ("维数大小"), 5 ("维数大小")) -> (w248:string[][])
      n407 = local write "Analog_back"(w248) -> ()
      n408 = local write "Analog_WC"(w248) -> ()
      n409 = local write "第几组数据"(w237) -> ()
      n410 = local write "第几个数据"(w237) -> ()
    }
  }
  n411 = Obtain Notifier(name (unnamed)=w8, notification data type=w8) -> (notifier out=w10:refnum<notifier>, error out=w9:errorcluster)  [unwired: 2 in, 1 out]
  n412 = while {
    tunnel: w10 -> [w377]
    tunnel: w9 -> [w376]
    tunnel: [w375] -> w7
    tunnel: [w374] -> w6
    stop <- w379 stop-if-true
    n413 = Wait Until Next ms Multiple(millisecond multiple=u32 10 ("毫秒倍数")) -> ()  [unwired: 1 out]
    n414 = Wait on Notification(notifier=w377, timeout in ms (-1)=20 ("超时毫秒(-1)"), error in (no error)=w376) -> (notifier out=w375:refnum<notifier>, notification=w383:string, error out=w374:errorcluster)  [unwired: 1 in, 1 out]
    n415 = Equal?(x=w383, y="DSP" ("通知")) -> (x = y?=w380:bool)
    n416 = case shown="真" w380 {
      frame False {
      }
      frame True {
        n417 = for {
          N: 16 -> [_]
          i -> [w388]
          n418 = local read "数组_选择"() -> (w391:bool[])
          n419 = disable-structure shown="禁用" {
            frame Disabled {
              n420 = property on="Analog_IN" class="Tbl (严格)"() -> ("Value"=w393:string[][])  [unwired: 2 in, 2 out]
              n421 = call "表格至数组.vi"("表格控件"=w393) -> ()  [unwired: 10 in, 1 out]
            }
            frame Enabled {
            }
          }
          n422 = local read "数组_设定值"() -> (w392:dbl[][])
          n423 = Add(x=w388, y=16) -> (x+y=w389:i32)
          n424 = Index Array(array=w391, index #1=w388, index #2=w389) -> (element #1=w386:bool, element #2=w385:bool)
          n425 = Or(x=w386, y=w385) -> (x .or. y?=w390:bool)
          n426 = case shown="真" w390 {
            tunnel: w388 -> [_ w394]
            tunnel: w392 -> [_ w396]
            frame False {
            }
            frame True {
              n427 = Increment(x=w394) -> (x+1=w397:i32)
              n428 = To Unsigned Byte Integer(number=w397) -> (unsigned 8bit integer=w398:u8)
              n429 = call "一组模拟量CAN切换开关.vi"("第几组数据"=w398) -> ()  [unwired: 10 in, 1 out]
              n430 = case shown="真" TRUE {
                tunnel: w394 -> [_ w399]
                tunnel: w396 -> [_ w400]
                frame False {
                }
                frame True {
                  n431 = local write "第几组数据"(w399) -> ()
                  n432 = for {
                    N: 5 -> [_]
                    tunnel: w399 -> [w404]
                    tunnel: w400 -> [w403]
                    i -> [w402]
                    n433 = while {
                      tunnel: w404 -> [w412]
                      tunnel: w403 -> [w411]
                      tunnel: w402 -> [w410]
                      stop <- w407 stop-if-true
                      n434 = local read "同步_1"() -> (w408:i32)
                      n435 = Wait Until Next ms Multiple(millisecond multiple=u32 10 ("毫秒倍数")) -> ()  [unwired: 1 out]
                      n436 = Equal?(x=w408, y=0) -> (x = y?=w409:bool)
                      n437 = case shown="真" w409 {
                        tunnel: w412 -> [_ w417]
                        tunnel: w411 -> [_ w416]
                        tunnel: w410 -> [_ w415]
                        tunnel: [FALSE w414] -> w407
                        frame False {
                        }
                        frame True {
                          n438 = stacked-sequence {
                            tunnel: w417 -> [_ w423 _ _ w441 _]
                            tunnel: w416 -> [_ w426 _ _ _ _]
                            tunnel: w415 -> [_ w419 _ _ _ _]
                            tunnel: [_ _ _ _ _ w442] -> w414
                            frame #0 {
                              n439 = Wait (ms)(milliseconds to wait=u32 100) -> ()  [unwired: 1 out]
                            }
                            frame #1 {
                              # "PCI板卡下发模拟量数据"
                              n440 = To Long Integer(number=w423) -> (32bit integer=w422:i32)
                              n441 = local write "第几个数据"(w419) -> ()
                              n442 = Add(x=w422, y=16) -> (x+y=w424:i32)
                              n443 = Index Array(array=w426, index (row) #1=w422, index (col) #1=w419, index (row) #2=w424, index (col) #2=w419) -> (element #1=w421:dbl, element #2=w420:dbl)
                              n444 = Build Array(w421, w420) -> (w427:dbl[])
                              n445 = call "Convert to Dynamic Data"("Array"=w427) -> ("Dynamic Data Type"=w428:dynamicdata)  [unwired: 3 out]
                              n446 = call "DAQNavi Assistant"("data in(DDT)"=w428) -> ()  [unwired: 2 in, 17 out]
                            }
                            frame #2 {
                              w431 = "ANumCheck" ("名称（未命名）")
                              n447 = Obtain Notifier(name (unnamed)=w431, notification data type=w431) -> (notifier out=w430:refnum<notifier>)  [unwired: 2 in, 2 out]
                              n448 = local write "同步_1"(1 ("同步_1")) -> ()
                              n449 = Send Notification(notification="NumCheck" ("通知"), notifier=w430) -> ()  [unwired: 1 in, 2 out]
                            }
                            frame #3 {
                              n450 = Wait (ms)(milliseconds to wait=u32 150) -> ()  [unwired: 1 out]
                            }
                            frame #4 {
                              # "待定"
                              # "待定"
                              # "待定"
                              # "以太网发送读取参数命令"
                              n451 = To Unsigned Word Integer(number=w441) -> (unsigned 16bit integer=w437:u16)
                              n452 = Add(x=w437, y=u16 16) -> (x+y=w438:u16)
                              n453 = Build Array(w437, w438) -> (w440:u16[])
                              n454 = call "UDP发送.vi"("发送数据"=w440, "数据区字长"=u16 2, "报文类型"=u16 2056, "发送方标识"=u16 5397) -> ()  [unwired: 6 in, 1 out]
                            }
                            frame #5 {
                              n455 = local read "同步_1"() -> (w444:i32)
                              n456 = Equal?(x=w444, y=1) -> (x = y?=w442:bool)
                            }
                          }
                        }
                      }
                    }
                  }
                }
              }
            }
          }
        }
      }
    }
    n457 = local read "退出？"() -> (w379:bool)
  }
  n458 = Release Notifier(notifier=w7, error in (no error)=w6) -> ()  [unwired: 1 in, 3 out]
  n459 = Obtain Notifier(name (unnamed)=w5, notification data type=w5) -> (notifier out=w4:refnum<notifier>, error out=w3:errorcluster)  [unwired: 2 in, 1 out]
  n460 = while {
    tunnel: w4 -> [w449]
    tunnel: w3 -> [w448]
    tunnel: [w447] -> w2
    tunnel: [w446] -> w1
    stop <- w445 stop-if-true
    n461 = Wait Until Next ms Multiple(millisecond multiple=u32 10 ("毫秒倍数")) -> ()  [unwired: 1 out]
    n462 = Wait on Notification(notifier=w449, timeout in ms (-1)=20 ("超时毫秒(-1)"), error in (no error)=w448) -> (notifier out=w447:refnum<notifier>, notification=w452:string, error out=w446:errorcluster)  [unwired: 1 in, 1 out]
    n463 = Equal?(x=w452, y="NumCheck" ("通知")) -> (x = y?=w450:bool)
    n464 = case shown="真" w450 {
      frame False {
      }
      frame True {
        w457 = u16 4
        w466 = u16 5397
        # "以太网返回查询到的参数"
        n465 = Build Array(w466, u16 2056, w457) -> (w463:u16[])
        n466 = Build Array(w466, u16 34952, u16 0 ("元素")) -> (w462:u16[])
        n467 = Add(x=w457, y=u16 4) -> (x+y=w455:u16)
        n468 = call "UDP接收.vi"("匹配帧信息_异常"=w462, "长度"=w455, "匹配帧信息_正常"=w463) -> ("异常_找到?"=w459:bool, "接收超时?"=w458:bool, "接收的一帧数据"=w460:u16[], "正常_找到?"=w461:bool)  [unwired: 5 in]
        n469 = case shown="真" w458 {
          frame False {
          }
          frame True {
            n470 = disable-structure shown="禁用" {
              frame Disabled {
                n471 = call "超时"() -> ()  [unwired: 10 in, 2 out]
              }
              frame Enabled {
              }
            }
            n472 = local write "同步_1"(0 ("同步_1")) -> ()
          }
        }
        n473 = case shown="真" w461 {
          tunnel: w460 -> [_ w476]
          frame False {
          }
          frame True {
            n474 = stacked-sequence {
              tunnel: w476 -> [w516 _ _ _]
              frame #0 {
                n475 = local read "第几组数据"() -> (w484:i32)
                n476 = local read "第几个数据"() -> (w479:i32)
                n477 = local read "数组_设定值"() -> (w510:dbl[][])
                n478 = local read "数组_选择"() -> (w488:bool[])
                n479 = Index Array(array=w516, index #1=3 ("索引"), index #2=4 ("索引"), index #3=5 ("索引"), index #4=6 ("索引")) -> (element #1=w495:u16, element #2=w494:u16, element #3=w493:u16, element #4=w492:u16)
                n480 = local read "第几组数据"() -> (w491:i32)
                n481 = Add(x=w484, y=16) -> (x+y=w497:i32)
                n482 = call "U16转换为float.vi"("第几组数据"=w491, "选择?"=w488, "低16位_2"=w492, "高16位_2"=w493, "低16位_1"=w494, "高16位_1"=w495) -> ("反馈值2"=w486:dbl, "反馈值1"=w477:dbl, "反馈值字符_2"=w489:string, "反馈值字符_1"=w490:string)  [unwired: 2 in]
                n483 = Index Array(array=w510, index (row) #1=w484, index (col) #1=w479, index (row) #2=w497, index (col) #2=w479) -> (element #1=w478:dbl, element #2=w485:dbl)
                n484 = local read "Analog_back"() -> (w502:string[][])
                n485 = local read "第几个数据"() -> (w496:i32)
                n486 = local read "数组_选择"() -> (w487:bool[])
                n487 = Add(x=w491, y=16) -> (x+y=w500:i32)
                n488 = call "一个反馈计算误差.vi"("第几组"=w484, "选择?"=w487, "设定值_2"=w485, "设定值_1"=w478, "反馈值_2"=w486, "反馈值_1"=w477) -> ("字符串_误差_2"=w481:string, "字符串_误差_1"=w482:string, "合格_2?"=w480:bool, "合格_1?"=w483:bool)  [unwired: 2 out]
                n489 = Replace Array Subset(array=w502, new element #1=w490, index (row) #1=w491, index (col) #1=w496, new element #2=w489, index (row) #2=w500, index (col) #2=w496) -> (w501:string[][])
                n490 = local write "Analog_back"(w501) -> ()
                n491 = local read "第几个数据"() -> (w498:i32)
                n492 = local read "Analog_WC"() -> (w507:string[][])
                n493 = local read "第几组数据"() -> (w505:i32)
                n494 = Add(x=w505, y=16) -> (x+y=w499:i32)
                n495 = Replace Array Subset(array=w507, new element #1=w482, index (row) #1=w505, index (col) #1=w498, new element #2=w481, index (row) #2=w499, index (col) #2=w498) -> (w506:string[][])
                n496 = local read "合格？"() -> (w503:bool[][])
                n497 = local write "Analog_WC"(w506) -> ()
                n498 = Replace Array Subset(array=w503, new element #1=w483, index (row) #1=w505, index (col) #1=w498, new element #2=w480, index (row) #2=w499, index (col) #2=w498) -> (w504:bool[][])
                n499 = local write "合格？"(w504) -> ()
              }
              frame #1 {
                n500 = local read "合格？"() -> (w526:bool[][])
                n501 = local read "第几组数据"() -> (w520:i32)
                n502 = Add(x=w520, y=16) -> (x+y=w519:i32)
                n503 = Index Array(array=w526, index (row) #1=w520, index (row) #2=w519) -> (element #1=w529:bool[], element #2=w523:bool[])  [unwired: 2 in]
                n504 = And Array Elements(Boolean array=w529) -> (logical AND=w524:bool)
                n505 = And Array Elements(Boolean array=w523) -> (logical AND=w522:bool)
                n506 = local read "数组_选择"() -> (w521:bool[])
                n507 = Index Array(array=w521, index #1=w520, index #2=w519) -> (element #1=w518:bool, element #2=w517:bool)
                n508 = case shown="真" w518 {
                  tunnel: [cluster{u32, u32}[] [{12369084, 12369084}] w537] -> w528
                  tunnel: w524 -> [_ w536]
                  frame False {
                  }
                  frame True {
                    n509 = case shown="真" w536 {
                      tunnel: [cluster{u32, u32}[] [{16730410, 16711680}] cluster{u32, u32}[] [{61205, 6618880}]] -> w537
                      frame False {
                      }
                      frame True {
                      }
                    }
                  }
                }
                n510 = case shown="真" w517 {
                  tunnel: [cluster{u32, u32}[] [{12369084, 12369084}] w532] -> w525
                  tunnel: w522 -> [_ w531]
                  frame False {
                  }
                  frame True {
                    n511 = case shown="真" w531 {
                      tunnel: [cluster{u32, u32}[] [{16730410, 16711680}] cluster{u32, u32}[] [{61205, 6618880}]] -> w532
                      frame False {
                      }
                      frame True {
                      }
                    }
                  }
                }
                n512 = case shown="31" w520 {
                  tunnel: w528 -> [w572 w573 w574 w575 w576 w577 w578 w579 w580 w581 w582 w583 w584 w585 w586 w587 w588 w589 w590 w591 w592 w593 w594 w595 w596 w597 w598 w599 w600 w601 w602 w603]
                  frame 0, Default {
                    n513 = property on="light_1" class="Bool (严格)"("Colors [4]"=w572) -> ()  [unwired: 2 in, 2 out]
                  }
                  frame 1 {
                    n514 = property on="light_2" class="Bool (严格)"("Colors [4]"=w573) -> ()  [unwired: 2 in, 2 out]
                  }
                  frame 2 {
                    n515 = property on="light_3" class="Bool (严格)"("Colors [4]"=w574) -> ()  [unwired: 2 in, 2 out]
                  }
                  frame 3 {
                    n516 = property on="light_4" class="Bool (严格)"("Colors [4]"=w575) -> ()  [unwired: 2 in, 2 out]
                  }
                  frame 4 {
                    n517 = property on="light_5" class="Bool (严格)"("Colors [4]"=w576) -> ()  [unwired: 2 in, 2 out]
                  }
                  frame 5 {
                    n518 = property on="light_6" class="Bool (严格)"("Colors [4]"=w577) -> ()  [unwired: 2 in, 2 out]
                  }
                  frame 6 {
                    n519 = property on="light_7" class="Bool (严格)"("Colors [4]"=w578) -> ()  [unwired: 2 in, 2 out]
                  }
                  frame 7 {
                    n520 = property on="light_8" class="Bool (严格)"("Colors [4]"=w579) -> ()  [unwired: 2 in, 2 out]
                  }
                  frame 8 {
                    n521 = property on="light_9" class="Bool (严格)"("Colors [4]"=w580) -> ()  [unwired: 2 in, 2 out]
                  }
                  frame 9 {
                    n522 = property on="light_10" class="Bool (严格)"("Colors [4]"=w581) -> ()  [unwired: 2 in, 2 out]
                  }
                  frame 10 {
                    n523 = property on="light_11" class="Bool (严格)"("Colors [4]"=w582) -> ()  [unwired: 2 in, 2 out]
                  }
                  frame 11 {
                    n524 = property on="light_12" class="Bool (严格)"("Colors [4]"=w583) -> ()  [unwired: 2 in, 2 out]
                  }
                  frame 12 {
                    n525 = property on="light_13" class="Bool (严格)"("Colors [4]"=w584) -> ()  [unwired: 2 in, 2 out]
                  }
                  frame 13 {
                    n526 = property on="light_14" class="Bool (严格)"("Colors [4]"=w585) -> ()  [unwired: 2 in, 2 out]
                  }
                  frame 14 {
                    n527 = property on="light_15" class="Bool (严格)"("Colors [4]"=w586) -> ()  [unwired: 2 in, 2 out]
                  }
                  frame 15 {
                    n528 = property on="light_16" class="Bool (严格)"("Colors [4]"=w587) -> ()  [unwired: 2 in, 2 out]
                  }
                  frame 16 {
                    n529 = property on="light_17" class="Bool (严格)"("Colors [4]"=w588) -> ()  [unwired: 2 in, 2 out]
                  }
                  frame 17 {
                    n530 = property on="light_18" class="Bool (严格)"("Colors [4]"=w589) -> ()  [unwired: 2 in, 2 out]
                  }
                  frame 18 {
                    n531 = property on="light_19" class="Bool (严格)"("Colors [4]"=w590) -> ()  [unwired: 2 in, 2 out]
                  }
                  frame 19 {
                    n532 = property on="light_20" class="Bool (严格)"("Colors [4]"=w591) -> ()  [unwired: 2 in, 2 out]
                  }
                  frame 20 {
                    n533 = property on="light_21" class="Bool (严格)"("Colors [4]"=w592) -> ()  [unwired: 2 in, 2 out]
                  }
                  frame 21 {
                    n534 = property on="light_22" class="Bool (严格)"("Colors [4]"=w593) -> ()  [unwired: 2 in, 2 out]
                  }
                  frame 22 {
                    n535 = property on="light_23" class="Bool (严格)"("Colors [4]"=w594) -> ()  [unwired: 2 in, 2 out]
                  }
                  frame 23 {
                    n536 = property on="light_24" class="Bool (严格)"("Colors [4]"=w595) -> ()  [unwired: 2 in, 2 out]
                  }
                  frame 24 {
                    n537 = property on="light_25" class="Bool (严格)"("Colors [4]"=w596) -> ()  [unwired: 2 in, 2 out]
                  }
                  frame 25 {
                    n538 = property on="light_26" class="Bool (严格)"("Colors [4]"=w597) -> ()  [unwired: 2 in, 2 out]
                  }
                  frame 26 {
                    n539 = property on="light_27" class="Bool (严格)"("Colors [4]"=w598) -> ()  [unwired: 2 in, 2 out]
                  }
                  frame 27 {
                    n540 = property on="light_28" class="Bool (严格)"("Colors [4]"=w599) -> ()  [unwired: 2 in, 2 out]
                  }
                  frame 28 {
                    n541 = property on="light_29" class="Bool (严格)"("Colors [4]"=w600) -> ()  [unwired: 2 in, 2 out]
                  }
                  frame 29 {
                    n542 = property on="light_30" class="Bool (严格)"("Colors [4]"=w601) -> ()  [unwired: 2 in, 2 out]
                  }
                  frame 30 {
                    n543 = property on="light_31" class="Bool (严格)"("Colors [4]"=w602) -> ()  [unwired: 2 in, 2 out]
                  }
                  frame 31 {
                    n544 = property on="light_32" class="Bool (严格)"("Colors [4]"=w603) -> ()  [unwired: 2 in, 2 out]
                  }
                }
                n545 = case shown="31" w519 {
                  tunnel: w525 -> [w540 w541 w542 w543 w544 w545 w546 w547 w548 w549 w550 w551 w552 w553 w554 w555 w556 w557 w558 w559 w560 w561 w562 w563 w564 w565 w566 w567 w568 w569 w570 w571]
                  frame 0, Default {
                    n546 = property on="light_1" class="Bool (严格)"("Colors [4]"=w540) -> ()  [unwired: 2 in, 2 out]
                  }
                  frame 1 {
                    n547 = property on="light_2" class="Bool (严格)"("Colors [4]"=w541) -> ()  [unwired: 2 in, 2 out]
                  }
                  frame 2 {
                    n548 = property on="light_3" class="Bool (严格)"("Colors [4]"=w542) -> ()  [unwired: 2 in, 2 out]
                  }
                  frame 3 {
                    n549 = property on="light_4" class="Bool (严格)"("Colors [4]"=w543) -> ()  [unwired: 2 in, 2 out]
                  }
                  frame 4 {
                    n550 = property on="light_5" class="Bool (严格)"("Colors [4]"=w544) -> ()  [unwired: 2 in, 2 out]
                  }
                  frame 5 {
                    n551 = property on="light_6" class="Bool (严格)"("Colors [4]"=w545) -> ()  [unwired: 2 in, 2 out]
                  }
                  frame 6 {
                    n552 = property on="light_7" class="Bool (严格)"("Colors [4]"=w546) -> ()  [unwired: 2 in, 2 out]
                  }
                  frame 7 {
                    n553 = property on="light_8" class="Bool (严格)"("Colors [4]"=w547) -> ()  [unwired: 2 in, 2 out]
                  }
                  frame 8 {
                    n554 = property on="light_9" class="Bool (严格)"("Colors [4]"=w548) -> ()  [unwired: 2 in, 2 out]
                  }
                  frame 9 {
                    n555 = property on="light_10" class="Bool (严格)"("Colors [4]"=w549) -> ()  [unwired: 2 in, 2 out]
                  }
                  frame 10 {
                    n556 = property on="light_11" class="Bool (严格)"("Colors [4]"=w550) -> ()  [unwired: 2 in, 2 out]
                  }
                  frame 11 {
                    n557 = property on="light_12" class="Bool (严格)"("Colors [4]"=w551) -> ()  [unwired: 2 in, 2 out]
                  }
                  frame 12 {
                    n558 = property on="light_13" class="Bool (严格)"("Colors [4]"=w552) -> ()  [unwired: 2 in, 2 out]
                  }
                  frame 13 {
                    n559 = property on="light_14" class="Bool (严格)"("Colors [4]"=w553) -> ()  [unwired: 2 in, 2 out]
                  }
                  frame 14 {
                    n560 = property on="light_15" class="Bool (严格)"("Colors [4]"=w554) -> ()  [unwired: 2 in, 2 out]
                  }
                  frame 15 {
                    n561 = property on="light_16" class="Bool (严格)"("Colors [4]"=w555) -> ()  [unwired: 2 in, 2 out]
                  }
                  frame 16 {
                    n562 = property on="light_17" class="Bool (严格)"("Colors [4]"=w556) -> ()  [unwired: 2 in, 2 out]
                  }
                  frame 17 {
                    n563 = property on="light_18" class="Bool (严格)"("Colors [4]"=w557) -> ()  [unwired: 2 in, 2 out]
                  }
                  frame 18 {
                    n564 = property on="light_19" class="Bool (严格)"("Colors [4]"=w558) -> ()  [unwired: 2 in, 2 out]
                  }
                  frame 19 {
                    n565 = property on="light_20" class="Bool (严格)"("Colors [4]"=w559) -> ()  [unwired: 2 in, 2 out]
                  }
                  frame 20 {
                    n566 = property on="light_21" class="Bool (严格)"("Colors [4]"=w560) -> ()  [unwired: 2 in, 2 out]
                  }
                  frame 21 {
                    n567 = property on="light_22" class="Bool (严格)"("Colors [4]"=w561) -> ()  [unwired: 2 in, 2 out]
                  }
                  frame 22 {
                    n568 = property on="light_23" class="Bool (严格)"("Colors [4]"=w562) -> ()  [unwired: 2 in, 2 out]
                  }
                  frame 23 {
                    n569 = property on="light_24" class="Bool (严格)"("Colors [4]"=w563) -> ()  [unwired: 2 in, 2 out]
                  }
                  frame 24 {
                    n570 = property on="light_25" class="Bool (严格)"("Colors [4]"=w564) -> ()  [unwired: 2 in, 2 out]
                  }
                  frame 25 {
                    n571 = property on="light_26" class="Bool (严格)"("Colors [4]"=w565) -> ()  [unwired: 2 in, 2 out]
                  }
                  frame 26 {
                    n572 = property on="light_27" class="Bool (严格)"("Colors [4]"=w566) -> ()  [unwired: 2 in, 2 out]
                  }
                  frame 27 {
                    n573 = property on="light_28" class="Bool (严格)"("Colors [4]"=w567) -> ()  [unwired: 2 in, 2 out]
                  }
                  frame 28 {
                    n574 = property on="light_29" class="Bool (严格)"("Colors [4]"=w568) -> ()  [unwired: 2 in, 2 out]
                  }
                  frame 29 {
                    n575 = property on="light_30" class="Bool (严格)"("Colors [4]"=w569) -> ()  [unwired: 2 in, 2 out]
                  }
                  frame 30 {
                    n576 = property on="light_31" class="Bool (严格)"("Colors [4]"=w570) -> ()  [unwired: 2 in, 2 out]
                  }
                  frame 31 {
                    n577 = property on="light_32" class="Bool (严格)"("Colors [4]"=w571) -> ()  [unwired: 2 in, 2 out]
                  }
                }
              }
              frame #2 {
                n578 = local read "第几组数据"() -> (w607:i32)
                n579 = Add(x=w607, y=16) -> (x+y=w609:i32)
                n580 = local read "第几个数据"() -> (w611:i32)
                n581 = local read "合格？"() -> (w612:bool[][])
                n582 = local read "数组_选择"() -> (w610:bool[])
                n583 = Index Array(array=w612, index (row) #1=w607, index (col) #1=w611, index (row) #2=w609, index (col) #2=w611) -> (element #1=w608:bool, element #2=w604:bool)
                n584 = Index Array(array=w610, index #1=w607, index #2=w609) -> (element #1=w606:bool, element #2=w605:bool)
                n585 = case shown="真" w606 {
                  tunnel: w611 -> [_ w623]
                  tunnel: w608 -> [_ w622]
                  tunnel: w607 -> [_ w621]
                  frame False {
                  }
                  frame True {
                    n586 = call "误差表格颜色.vi"("合格？"=w622, "第几组"=w621) -> ("颜色"=w620:u32)  [unwired: 9 in]
                    n587 = Bundle("第几组数据"=w621, "第几个数据"=w623) -> (w625:cluster{"第几组数据":i32, "第几个数据":i32})  [unwired: 1 in]
                    n588 = property on="Analog_WC" class="Tbl (严格)"("Active Cell"=w625) -> (error out=w624:errorcluster)  [unwired: 2 in, 1 out]
                    n589 = property on="Analog_WC" class="Tbl (严格)"(error in=w624, "Cell BG Color"=w620) -> ()  [unwired: 1 in, 2 out]
                  }
                }
                n590 = case shown="真" w605 {
                  tunnel: w611 -> [_ w617]
                  tunnel: w609 -> [_ w616]
                  tunnel: w604 -> [_ w614]
                  frame False {
                  }
                  frame True {
                    n591 = Bundle(w616, "第几个数据"=w617) -> (w618:cluster{i32, "第几个数据":i32})  [unwired: 1 in]
                    n592 = call "误差表格颜色.vi"("合格？"=w614, "第几组"=w616) -> ("颜色"=w615:u32)  [unwired: 9 in]
                    n593 = property on="Analog_WC" class="Tbl (严格)"("Active Cell"=w618) -> (error out=w619:errorcluster)  [unwired: 2 in, 1 out]
                    n594 = property on="Analog_WC" class="Tbl (严格)"(error in=w619, "Cell BG Color"=w615) -> ()  [unwired: 1 in, 2 out]
                  }
                }
              }
              frame #3 {
                n595 = flat-sequence {
                  frame #0 {
                    n596 = Wait Until Next ms Multiple(millisecond multiple=u32 100) -> ()  [unwired: 1 out]
                  }
                  frame #1 {
                    n597 = local write "同步_1"(0 ("同步_1")) -> ()
                  }
                }
              }
            }
          }
        }
        n598 = case shown="真" w459 {
          frame False {
          }
          frame True {
            # "第几个"
            # "第几组"
            n599 = local read "第几个数据"() -> (w470:i32)
            n600 = local read "第几组数据"() -> (w472:i32)
            n601 = Increment(x=w472) -> (x+1=w473:i32)
            n602 = Increment(x=w470) -> (x+1=w471:i32)
            n603 = Format Into String(format string="第%d组%d个数据反馈失败（UDP）" ("Message"), w473, w471) -> (resulting string=w474:string)  [unwired: 2 in, 1 out]
            n604 = call "显示对话框信息2"("Message"=w474) -> ()  [unwired: 9 in, 2 out]
            n605 = local write "同步_1"(0 ("同步_1")) -> ()
          }
        }
      }
    }
    n606 = local read "退出？"() -> (w445:bool)
  }
  n607 = Release Notifier(notifier=w2, error in (no error)=w1) -> ()  [unwired: 1 in, 3 out]
